vi "DrawCross.vi"(8 "color":u32(colorbox)=6618880, 9 "pixel":i32, 10 "position":cluster{"x":i16, "y":i16}, 11 "picture input":picture) -> (3 "picture Output":picture)   [LabVIEW 2011]
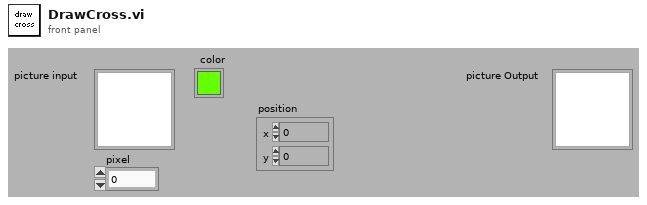
[diagram p1: front panel]
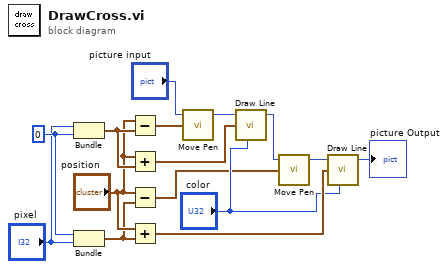
[diagram p0: block diagram]
diagram:
  w14 = 0
  n1 = Bundle("pixel"="pixel", w14) -> (w12:cluster{"pixel":i32, i32})  [unwired: 1 out]
  n2 = Bundle(w14, "pixel"="pixel") -> (w10:cluster{i32, "pixel":i32})  [unwired: 1 out]
  n3 = Subtract(x="position", y=w12) -> (x-y=w5:cluster{i32, i32})
  n4 = Add(x="position", y=w12) -> (x+y=w15:cluster{i32, i32})
  n5 = Subtract(x="position", y=w10) -> (x-y=w3:cluster{i32, i32})
  n6 = Add(x="position", y=w10) -> (x+y=w9:cluster{i32, i32})
  n7 = call <vilib>:"Move Pen.vi"("new position"=w5, "picture"="picture input") -> ("new picture"=w4:picture)  [unwired: 1 in, 2 out]
  n8 = call <vilib>:"Draw Line.vi"("picture"=w4, "end point"=w15, "color(black)"="color") -> ("new picture"=w2:picture)  [unwired: 2 in, 4 out]
  n9 = call <vilib>:"Move Pen.vi"("new position"=w3, "picture"=w2) -> ("new picture"=w1:picture)  [unwired: 1 in, 2 out]
  n10 = call <vilib>:"Draw Line.vi"("picture"=w1, "end point"=w9, "color(black)"="color") -> ("new picture"=→"picture Output":picture)  [unwired: 2 in, 4 out]
